vi "Vision Processing.vi"(4 "error in (no error)":errorcluster, 5 "Camera Type":enum16{"206", "1011"}(ring), 6 "Camera Name":string="Camera") -> ()   [LabVIEW 2011]
uses:
  Robot Global Data.vi
  <vilib>/vision/NI_Vision_Development_Module.lvlib
panel:
  in  "View":bool
  out "Target Info":T1(array[cluster])
  in  "Area Size Limit":i32=444
  in  "Particle Count Limit":i32=8
  in  "Score Limits":T2={"Rect Coverage"=76.0, "Aspect Ratio"=70.0, "X Edge Strength"=40.0, "Y Edge Strength"=60.0}
  in  "Processing":enum32{"Color", "Intensity", "Intensity Open"}(tab)
  in  "Range":cluster{"Lower value":sgl, "Upper value":sgl}={"Lower value"=150.0, "Upper value"=255.0} {"Lower value" scale=0.0..255.0; "Upper value" scale=0.0..255.0}
  in  "Range":cluster{"Lower value":sgl, "Upper value":sgl}={"Lower value"=150.0, "Upper value"=255.0} {"Lower value" scale=0.0..255.0; "Upper value" scale=0.0..255.0}
  in  "View":bool
  out "Processed Image":T3(plugin-control)
  out "Original Image":T3(plugin-control)
  # "Instructions:\nProcessing the reflective tape that is illuminated by a ring light can be based\non color or light intensity.\nParticles within the image are scored by rectangle coverage, aspect ratio, and\nfor being hollow with a bold edge. A particle is considered a target if all scores\nare above the score limits. Particles can be annotated -- surrounded by\na rectangle and scores drawn to the left .\nTo control the number of particles being scored, use the count limit and the size\nlimit."
  # "To debug, Enable using the View button.\nFor color processing, you can click in the image to select the color for processing."
  # "Enable by clicking the View button.\nGreen scores are above the limit, orange are below. Inner/outer rect\nindicates all passed."
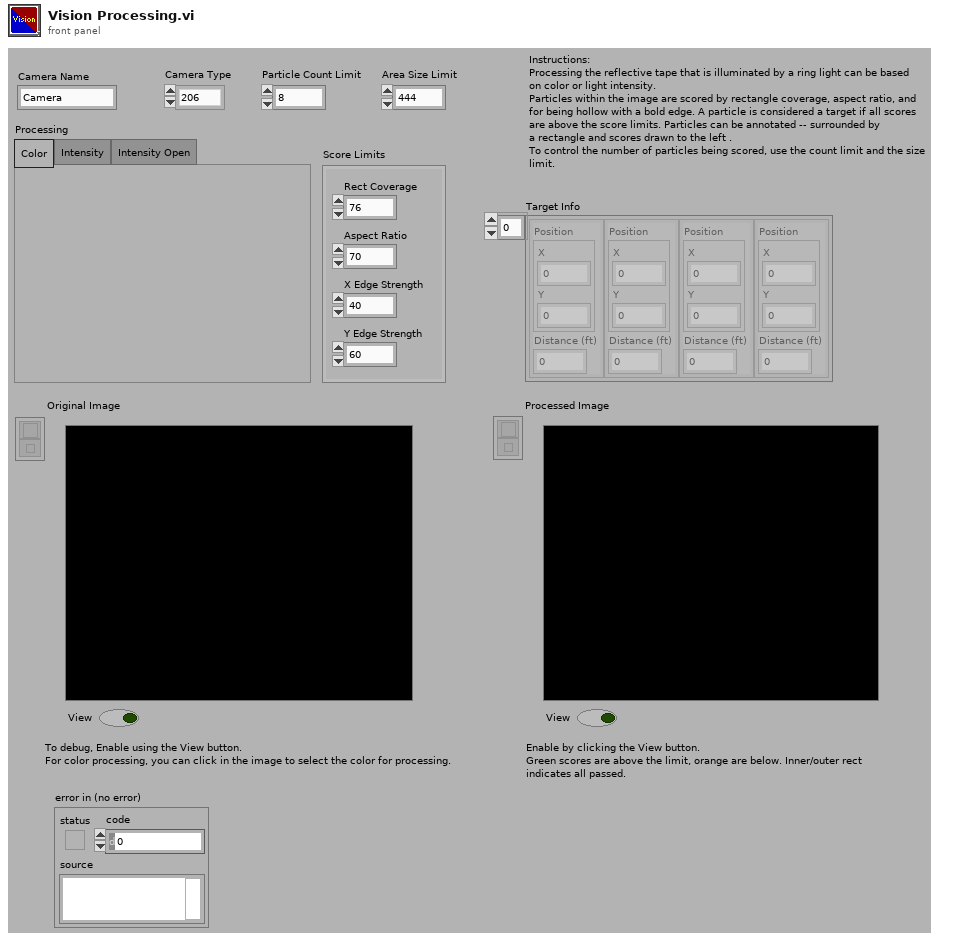
[diagram p1: front panel]
types:
  T1 = cluster{"Position":cluster{"X":dbl, "Y":dbl}, "Distance (ft)":dbl}[]
  T2 = cluster{"Rect Coverage":dbl, "Aspect Ratio":dbl, "X Edge Strength":dbl, "Y Edge Strength":dbl}
  T3 = typedef "IMAQ Image.ctl" = refnum<image>
  T4 = typedef "Image Type" = u32
  T5 = typedef "WPI_CameraDevRef.ctl" = cluster{"Camera Address":string, "CameraStatus":errorcluster, "Acquire Image Notifier":refnum<notifier>}
  T6 = enum32{"AutoM", "Close", "Dilate", "Erode", "Gradient", "Gradient out", "Gradient in", "Hit miss", "Open", "PClose", "POpen", "Thick", "Thin"}
  T7 = typedef "WPI_CameraImageSize.ctl" = enum16{"640x480", "320x240", "160x120"}
  T8 = cluster{cluster{"Left":dbl, "Top":dbl, "Right":dbl, "Bottom":dbl}, dbl[]}[]
  T9 = cluster{"Left":dbl, "Top":dbl, "Right":dbl, "Bottom":dbl}
  T10 = cluster{"Target Center (-1 to 1)":cluster{"X":dbl, "Y":dbl}, "Distance (ft)":dbl}
  T11 = cluster{"Target Center (-1 to 1)":cluster{"X":dbl, "Y":dbl}, "Distance (ft)":dbl}[]
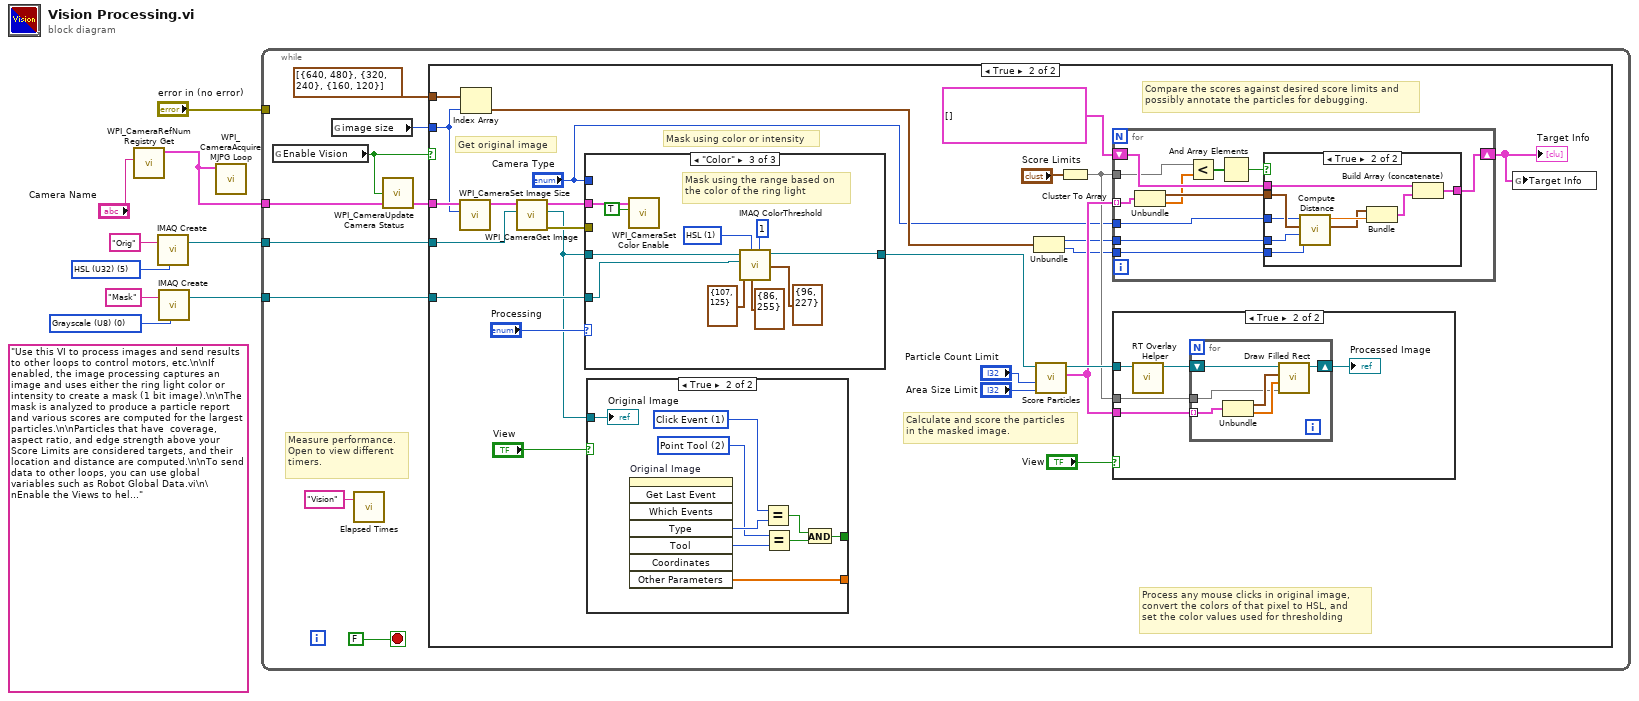
[diagram p0: block diagram]
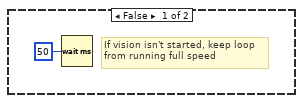
[diagram p2: hidden frame]
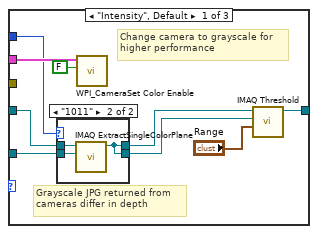
[diagram p3: hidden frame]
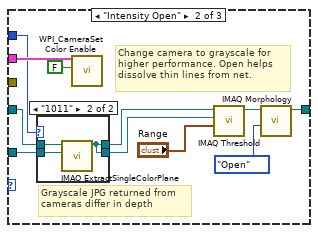
[diagram p5: hidden frame]
diagram:
  w3 = T4 0 items=["Grayscale (U8)", "Grayscale (I16)", "Grayscale (SGL)", "Complex (CSG)", "RGB (U32)", "HSL (U32)", "RGB (U64)", "Grayscale (U16)"] ("Image Type")
  (unwired) "Use this VI to process images and send results to other loops to control motors, etc.\n\nIf enabled, the image processing captures an image and uses either the ring light color or intensity to create a mask (1 bit image).\n\nThe mask is analyzed to produce a particle report and various scores are computed for the largest particles.\n\nParticles that have  coverage, aspect ratio, and edge strength above your Score Limits are considered targets, and their location and distance are computed.\n\nTo send data to other loops, you can use global variables such as Robot Global Data.vi\n\nEnable the Views to help debug color settings. Disable the View to speed up processing."
  w8 = T4 5 items=["Grayscale (U8)", "Grayscale (I16)", "Grayscale (SGL)", "Complex (CSG)", "RGB (U32)", "HSL (U32)", "RGB (U64)", "Grayscale (U16)"] ("Image Type")
  n1 = call <vilib>:"WPI_CameraRefNum Registry Get.vi"("refnum name"="Camera Name") -> ("CameraDevRef"=w5:T5)  [unwired: 9 in, 1 out]
  n2 = call "IMAQ Create"("Image Name"="Orig", "Image Type"=w8) -> ("New Image"=w7:T3)  [unwired: 2 in, 2 out]
  n3 = call "IMAQ Create"("Image Name"="Mask", "Image Type"=w3) -> ("New Image"=w1:T3)  [unwired: 2 in, 2 out]
  n4 = call <vilib>:"WPI_CameraAcquire MJPG Loop.vi"("CameraDevRef"=w5) -> ()  [unwired: 11 in]
  n5 = while {
    tunnel: w7 -> [w17]
    tunnel: w5 -> [w16]
    tunnel: "error in (no error)" -> [_]
    tunnel: w1 -> [w11]
    stop <- FALSE stop-if-true
    # "Measure performance.\nOpen to view different\ntimers."
    n6 = global read "Robot Global Data.vi" "Enable Vision"() -> (w14:bool)
    n7 = global read "Robot Global Data.vi" "image size"() -> (w12:T7)
    n8 = call "Elapsed Times.vi"("Call Name"="Vision") -> ()  [unwired: 2 in, 1 out]
    n9 = call <vilib>:"WPI_CameraUpdate Camera Status.vi"("CameraDevRef In"=w16, "Enable Vision"=w14) -> ("CameraDevRef Out"=w15:T5)  [unwired: 3 in]
    n10 = case shown="True" w14 {
      tunnel: w17 -> [_ w35]
      tunnel: w15 -> [_ w30]
      tunnel: w12 -> [_ w27]
      tunnel: w11 -> [_ w22]
      tunnel: cluster{i32, i32}[] [{640, 480}, {320, 240}, {160, 120}] -> [_ w26]
      frame False {
        # "If vision isn't started, keep loop\nfrom running full speed"
        n11 = Wait (ms)(milliseconds to wait=u32 50) -> ()  [unwired: 1 out]
      }
      frame True {
        # "Compare the scores against desired score limits and\npossibly annotate the particles for debugging."
        # "Process any mouse clicks in original image,\nconvert the colors of that pixel to HSL, and\nset the color values used for thresholding"
        # "Calculate and score the particles\nin the masked image."
        # "Mask using color or intensity"
        # "Get original image"
        n12 = call <vilib>:"WPI_CameraSet Image Size.vi"("Image Size"=w27, "CameraDevRef"=w30) -> ("CameraDevRef Out"=w31:T5)  [unwired: 8 in, 1 out]
        n13 = Index Array(array=w26, index=w27) -> (element=w23:cluster{i32, i32})
        n14 = call <vilib>:"WPI_CameraGet Image.vi"("Image"=w35, "CameraDevRef"=w31) -> ("error out"=w33:errorcluster, "Image Out"=w21:T3, "CameraDevRef Out"=w34:T5)  [unwired: 7 in]
        n15 = case shown="\"Color\"" "Processing" {
          tunnel: w21 -> [w49 w61 w76]
          tunnel: [w52 w66 w75] -> w28
          tunnel: w34 -> [w50 w64 w84]
          tunnel: w33 -> [_ _ _]
          tunnel: w22 -> [w48 w62 w77]
          tunnel: "Camera Type" -> [w47 w63 _]
          frame "Intensity", Default {
            # "Grayscale JPG returned from\ncameras differ in depth"
            # "Change camera to grayscale for\nhigher performance"
            n16 = case shown="\"1011\"" w47 {
              tunnel: w49 -> [w55 w58]
              tunnel: w48 -> [w54 w57]
              tunnel: [w55 w56] -> w46
              tunnel: [w54 w56] -> w45
              frame "206", Default {
              }
              frame "1011" {
                n17 = call "IMAQ ExtractSingleColorPlane"("Image Dst"=w57, "Image Src"=w58) -> ("Image Dst Out"=w56:T3)  [unwired: 8 in, 1 out]
              }
            }
            n18 = call <vilib>:"WPI_CameraSet Color Enable.vi"("Color Enabled"=FALSE, "CameraDevRef"=w50) -> ()  [unwired: 8 in, 2 out]
            n19 = call "IMAQ Threshold"("Range"="Range", "Image Dst"=w45, "Image Src"=w46) -> ("Image Dst Out"=w52:T3)  [unwired: 3 in, 5 out]
          }
          frame "Intensity Open" {
            # "Grayscale JPG returned from\ncameras differ in depth"
            # "Change camera to grayscale for\nhigher performance. Open helps\ndissolve thin lines from net."
            n20 = case shown="\"1011\"" w63 {
              tunnel: w61 -> [w71 w74]
              tunnel: w62 -> [w70 w73]
              tunnel: [w71 w72] -> w60
              tunnel: [w70 w72] -> w59
              frame "206", Default {
              }
              frame "1011" {
                n21 = call "IMAQ ExtractSingleColorPlane"("Image Dst"=w73, "Image Src"=w74) -> ("Image Dst Out"=w72:T3)  [unwired: 8 in, 1 out]
              }
            }
            n22 = call <vilib>:"WPI_CameraSet Color Enable.vi"("Color Enabled"=FALSE, "CameraDevRef"=w64) -> ()  [unwired: 8 in, 2 out]
            n23 = call "IMAQ Threshold"("Range"="Range", "Image Dst"=w59, "Image Src"=w60) -> ("Image Dst Out"=w67:T3)  [unwired: 3 in, 5 out]
            n24 = call "IMAQ Morphology"("Operation"=T6."Open", "Image Src"=w67) -> ("Image Dst Out"=w66:T3)  [unwired: 8 in, 1 out]
          }
          frame "Color" {
            w80 = u16 1 items=["RGB", "HSL", "HSV", "HSI"] ("Color Mode")
            # "Mask using the range based on\nthe color of the ring light"
            n25 = call <vilib>:"WPI_CameraSet Color Enable.vi"("Color Enabled"=TRUE, "CameraDevRef"=w84) -> ()  [unwired: 8 in, 2 out]
            n26 = call "IMAQ ColorThreshold"("Blue or Luma or Val or Inten Range"=cluster{"Lower value":i32, "Upper value":i32} {"Lower value"=96, "Upper value"=227}, "Replace Value"=1, "Green or Sat Range"=cluster{"Lower value":i32, "Upper value":i32} {"Lower value"=86, "Upper value"=255}, "Color Mode"=w80, "Red or Hue Range"=cluster{"Lower value":i32, "Upper value":i32} {"Lower value"=107, "Upper value"=125}, "Image Dst"=w77, "Image Src"=w76) -> ("Image Dst Out"=w75:T3)  [unwired: 1 in, 3 out]
          }
        }
        n27 = case shown="True" "View" {
          tunnel: w21 -> [_ w104]
          tunnel: [_ w99] -> _
          tunnel: [_ w96] -> _
          frame False {
          }
          frame True {
            w97 = 2 items=["None", "Selection Tool", "Point Tool", "Line Tool", "Rectangle Tool", "Oval Tool", "Polygon Tool", "ClosedFreehandTool", "Annulus Tool", "Rotated Rectangle Tool", "Zoom Tool", "Pan Tool", "Polyline Tool", "Freehand Tool"] ("Tool")
            w98 = 1 items=["No Event"=0, "Click Event"=1, "Draw Event"=2, "Size Event"=4, "Scroll Event"=5, "Double Click Event"=8] ("Type")
            n28 = invoke on="Original Image" class="ImageControl" method="Get Last Event"() -> ("Type"=w100:i32, "Tool"=w103:i32, "Other Parameters"=w96:sgl[])  [unwired: 8 in, 5 out]
            n29 = Equal?(x=w98, y=w100) -> (x = y?=w101:bool)
            n30 = Equal?(x=w97, y=w103) -> (x = y?=w102:bool)
            n31 = And(x=w101, y=w102) -> (x .and. y?=w99:bool)
            "Original Image" <- w104
          }
        }
        n32 = Unbundle(w23) -> (w25:i32, w24:i32)
        n33 = call "Score Particles.vi"("Area Size Limit"="Area Size Limit", "Particle Count Limit"="Particle Count Limit", "Image Refnum in"=w28) -> ("Scored Particle Info"=w40:T8, "Image Refnum out"=w43:T3)  [unwired: 7 in]
        n34 = Cluster To Array(cluster="Score Limits") -> (array=w38:dbl[])
        n35 = for {
          shift-right: [w114] -> w32
          shift-left: T1 [] -> [w115]
          tunnel: w25 -> [w113]
          tunnel: w40 -> [w111] mode=indexing
          tunnel: w38 -> [w106]
          tunnel: "Camera Type" -> [w110]
          tunnel: w24 -> [w105]
          n36 = Unbundle(w111) -> (w112:T9, w107:dbl[])
          n37 = Less?(x=w106, y=w107) -> (x < y?=w109:bool[])
          n38 = And Array Elements(Boolean array=w109) -> (logical AND=w108:bool)
          n39 = case shown="True" w108 {
            tunnel: w115 -> [w116 w125]
            tunnel: [w116 w124] -> w114
            tunnel: w112 -> [_ w120]
            tunnel: w113 -> [_ w122]
            tunnel: w110 -> [_ w119]
            tunnel: w105 -> [_ w118]
            frame False {
            }
            frame True {
              n40 = call "Compute Distance.vi"("Y Image Resolution"=w118, "X Image Resolution"=w122, "Bounding Box"=w120, "Camera Type"=w119) -> ("Target Center (-1 to 1)"=w117:cluster{"X":dbl, "Y":dbl}, "Distance (ft)"=w121:dbl)  [unwired: 6 in]
              n41 = Bundle("Target Center (-1 to 1)"=w117, "Distance (ft)"=w121) -> (w123:T10)  [unwired: 1 in]
              n42 = Build Array (concatenate)(w125, w123) -> (w124:T11)
            }
          }
        }
        "Target Info" <- w32
        n43 = case shown="True" "View" {
          tunnel: w43 -> [_ w86]
          tunnel: w40 -> [_ w88]
          tunnel: w38 -> [_ w87]
          frame False {
          }
          frame True {
            n44 = call "RT Overlay Helper.vi"("Refnum in"=w86) -> ("Refnum out"=w89:T3)  [unwired: 10 in]
            n45 = for {
              shift-right: [w94] -> w85
              shift-left: w89 -> [w95]
              tunnel: w88 -> [w91] mode=indexing
              tunnel: w87 -> [w90]
              n46 = Unbundle(w91) -> (w92:T9, w93:dbl[])
              n47 = call "Draw Filled Rect.vi"("Limits"=w90, "Scores"=w93, "Bounding Box"=w92, "image in"=w95) -> ("image out"=w94:T3)  [unwired: 7 in]
            }
            "Processed Image" <- w85
          }
        }
        n48 = global write "Robot Global Data.vi" "Target Info"(w32) -> ()
      }
    }
  }
